vi "Simulation.SetAllObjectRefs.vi"(8 "error in (no error)":errorcluster, 11 "Simulation in":refnum<class "Simulation.lvclass">) -> (0 "error out":errorcluster, 3 "Simulation out":refnum<class "Simulation.lvclass">)   [LabVIEW 2016, in "Simulation.lvclass"]
uses:
  Simulation.lvclass
  Simulation.lvclass/Simulation.ctl
  Modell/Hausmodell/Hausmodell.lvclass
  Modell/Sondenmodell/Sondenmodell.lvclass
  Modell/Umgebung/Umgebung.lvclass
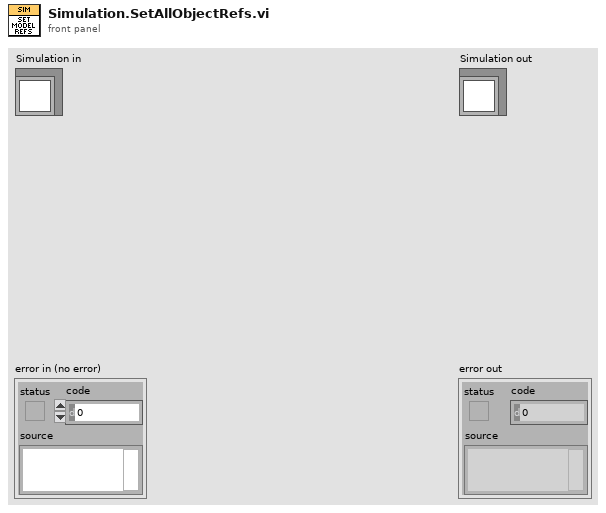
[diagram p1: front panel]
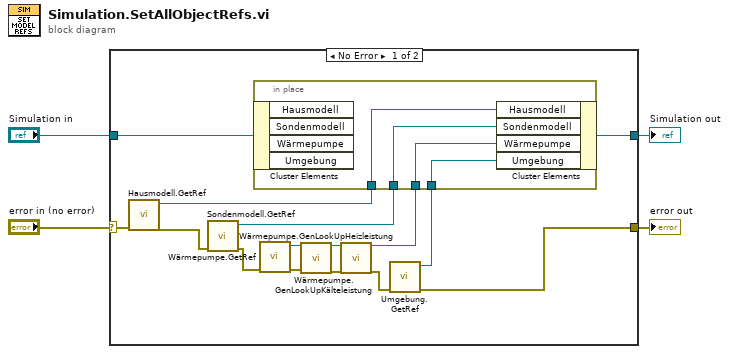
[diagram p0: block diagram]
diagram:
  n1 = case shown="No Error" "error in (no error)" {
    selector: "error in (no error)" -> [w19 w25]
    tunnel: [w11 w25] -> w3
    tunnel: [w13 w24] -> w1
    tunnel: "Simulation in" -> [w16 w24]
    frame No Error {
      n2 = call "Hausmodell.GetRef.vi"("Error In"=w19) -> ("Error out"=w18:errorcluster, "Hausmodell"=w15:refnum<data-value>)  [unwired: 9 in]
      n3 = call "Sondenmodell.GetRef.vi"("Error In"=w18) -> ("Error out"=w17:errorcluster, "Sondenmodell"=w14:refnum<data-value>)  [unwired: 9 in]
      n4 = call "Wärmepumpe.GetRef.vi"("Error In"=w17) -> ("Error out"=w7:errorcluster, "Wärmepumpe"=w12:refnum<data-value>)  [unwired: 9 in]
      n5 = call "Wärmepumpe.GenLookUpHeizleistung.vi"("Wärmepumpe in"=w12, "Error in"=w7) -> ("Wärmepumpe out"=w9:refnum<data-value>, "Error out"=w6:errorcluster)  [unwired: 16 in]
      n6 = call "Wärmepumpe.GenLookUpKälteleistung.vi"("Wärmepumpe in"=w9, "Error in"=w6) -> ("Wärmepumpe out"=w8:refnum<data-value>, "Error out"=w5:errorcluster)  [unwired: 16 in]
      n7 = call "Umgebung.GetRef.vi"("Error in"=w5) -> ("Error out"=w11:errorcluster, "Umgebung"=w10:refnum<data-value>)  [unwired: 9 in]
      n8 = in-place {
        in-place-border: w15 -> [w23]
        in-place-border: w14 -> [w22]
        in-place-border: w8 -> [w21]
        in-place-border: w10 -> [w20]
        n9 = in-place-cluster #1(w16) -> ()  [unwired: 4 out]
        n10 = in-place-cluster #1("Hausmodell"=w23, "Sondenmodell"=w22, "Wärmepumpe"=w21, "Umgebung"=w20) -> (w13:refnum<class "Simulation.lvclass">)
      }
    }
    frame Error {
    }
  }
  "error out" <- w3
  "Simulation out" <- w1
